vi "GUI Calibration AI.vi"(11 "error in":errorcluster) -> (15 "error out":errorcluster)   [LabVIEW 2019]
uses:
  TypeDef/CalbrationPoint.ctl
  TypeDef/GUI Setting Channel.ctl
  <vilib>/Analysis/NI_AALPro.lvlib
  <vilib>/Analysis/6fits.llb/Curve Fitting Criteria.ctl
panel:
  in  "Manual insert":bool caption="Ввод необработанного значений вручную"
  out "XY Graph - Dark":cluster{dbl[], dbl[]}[](graph) caption="Калибровачный график"
  in  "Current EU":dbl caption="Текущее значение вводится оператором"
  in  "Current RAW":dbl caption="Текущее необработанное значение"
  out "Offset":dbl caption="Смещение, EU"
  out "Коэфициент усиление":dbl caption="Коэфициент \nусиление EU/mA"
  in  "Remove Point":bool
  in  "Add Point":bool
  in  "Channels config":i32(listbox)
  in  "Channels":i32(listbox)
  # "Калибровка каналов"
  # "Параметры пересчета"
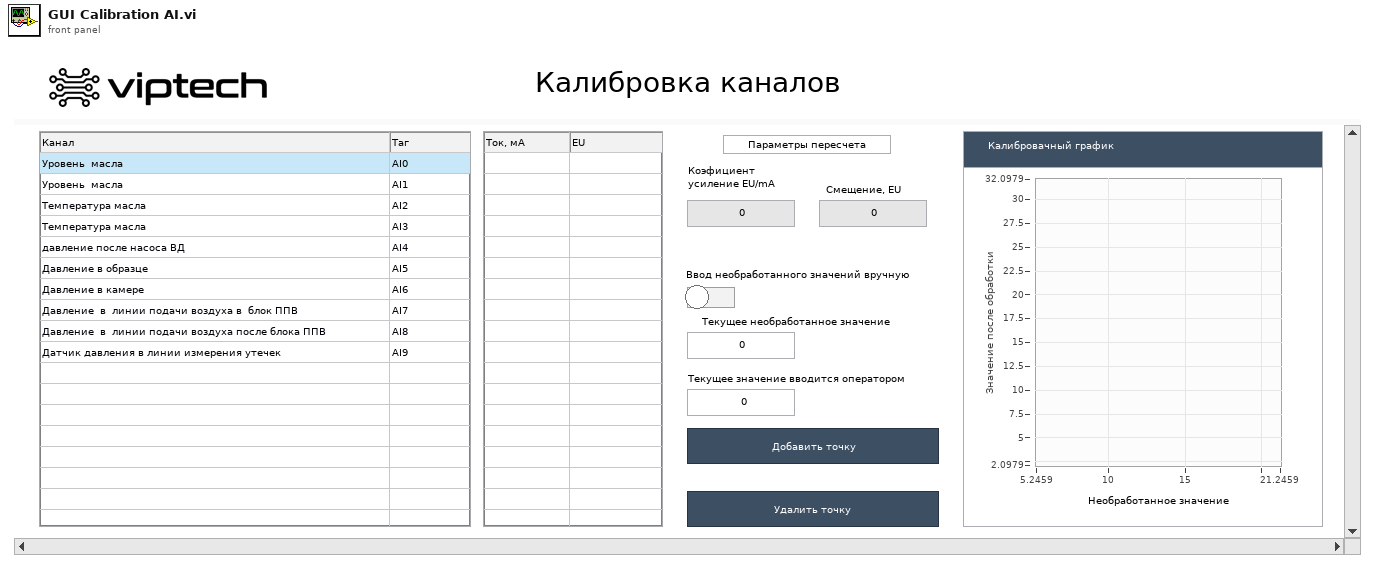
[diagram p1: front panel]
types:
  T1 = typedef "CalbrationPoint.ctl" = cluster{"RAW":dbl, "SCL":dbl}
  T2 = enum32{"Invalid", "Standard", "Closed", "Hidden", "Minimized", "Maximized"}
  T3 = enum32{"invalid app kind", "Development System", "Run Time System", "Student Edition", "Embedded LabVIEW", "Evaluation", "Custom"}
  T4 = typedef "GUI Setting Channel.ctl" = cluster{"Name":string, "SensorID":u32}
  T5 = cluster{"Core":cluster{"Current VI Reference":refnum<vi>, "Close Panel on Exit?":bool}, "Calibration Data":T4[], "Channels ref":refnum<vi>, "Channels config ref":refnum<vi>, "Channels config":i32, "Channels":i32}
  T6 = cluster{"Current VI Reference":refnum<vi>, "Close Panel on Exit?":bool}
  T7 = typedef "NI_AALPro.lvlib/Curve Fitting Criteria.ctl" = u16
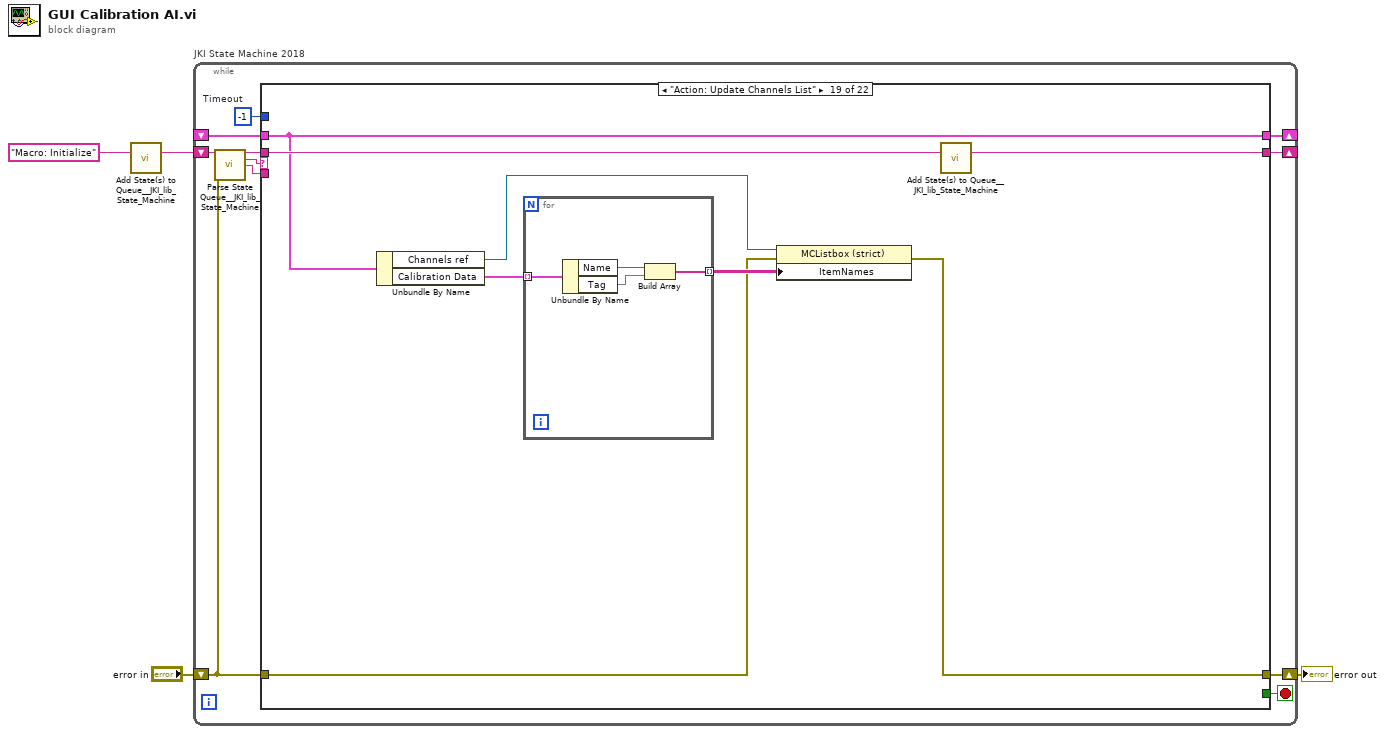
[diagram p0: block diagram]
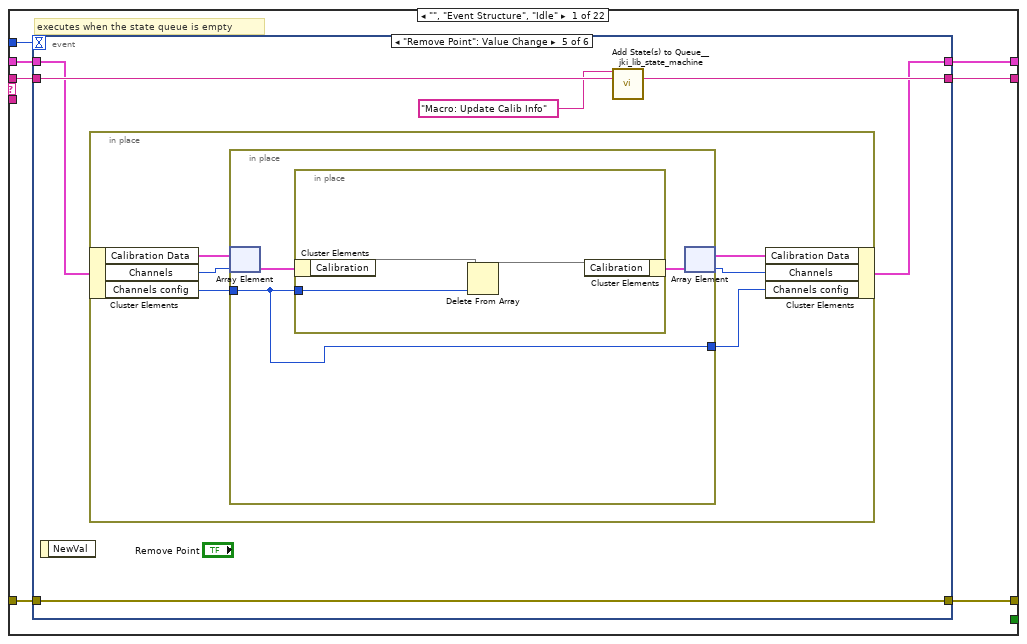
[diagram p2: hidden frame]
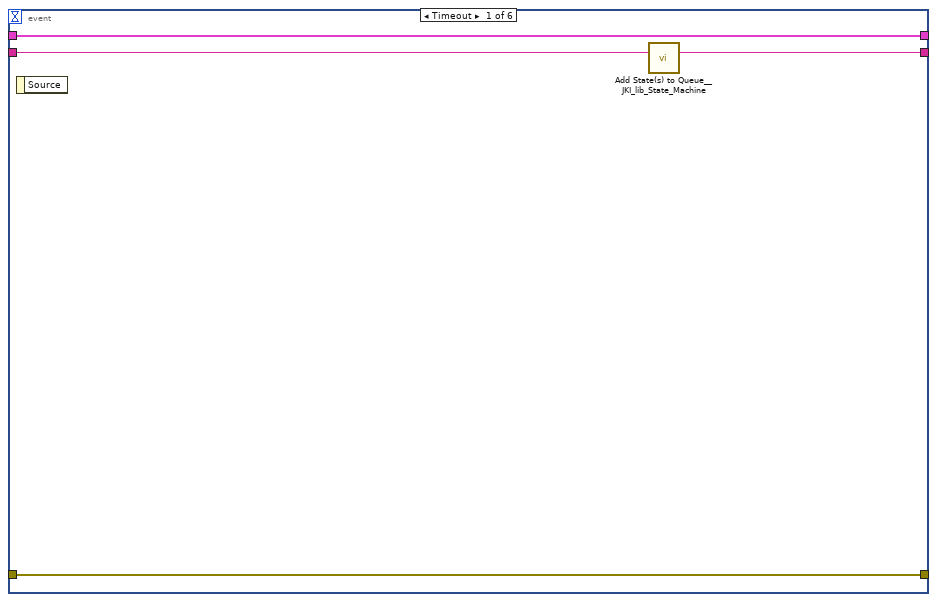
[diagram p3: hidden frame]
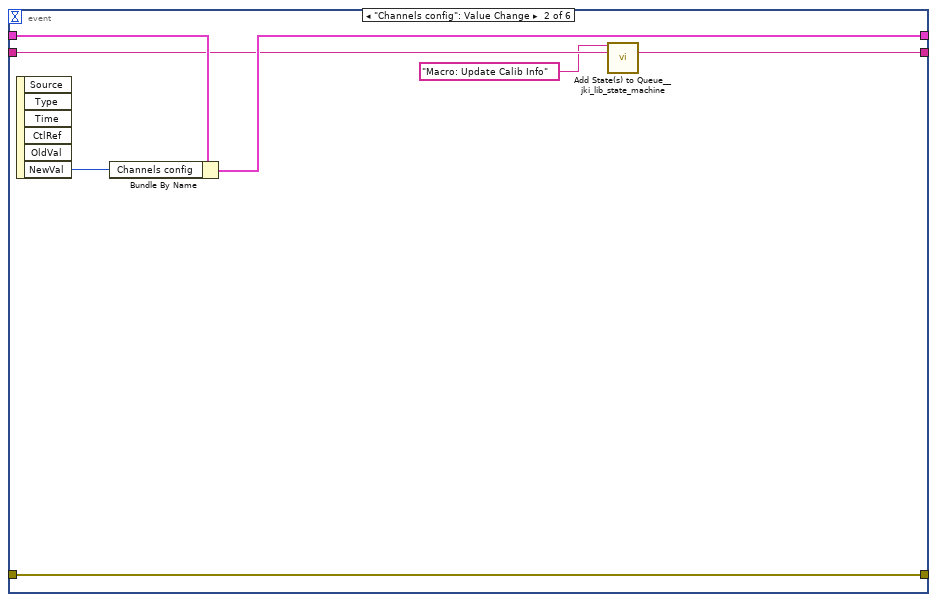
[diagram p4: hidden frame]
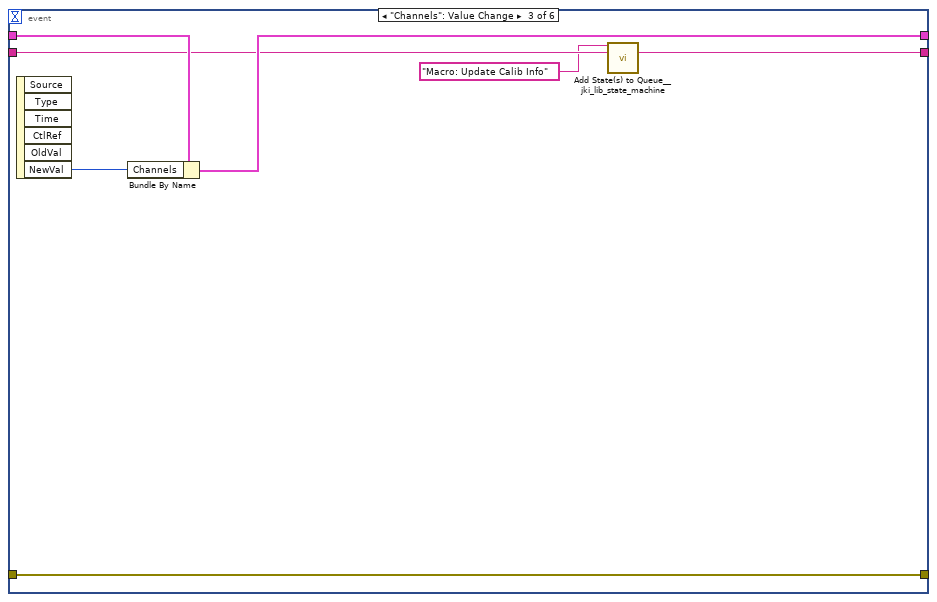
[diagram p5: hidden frame]
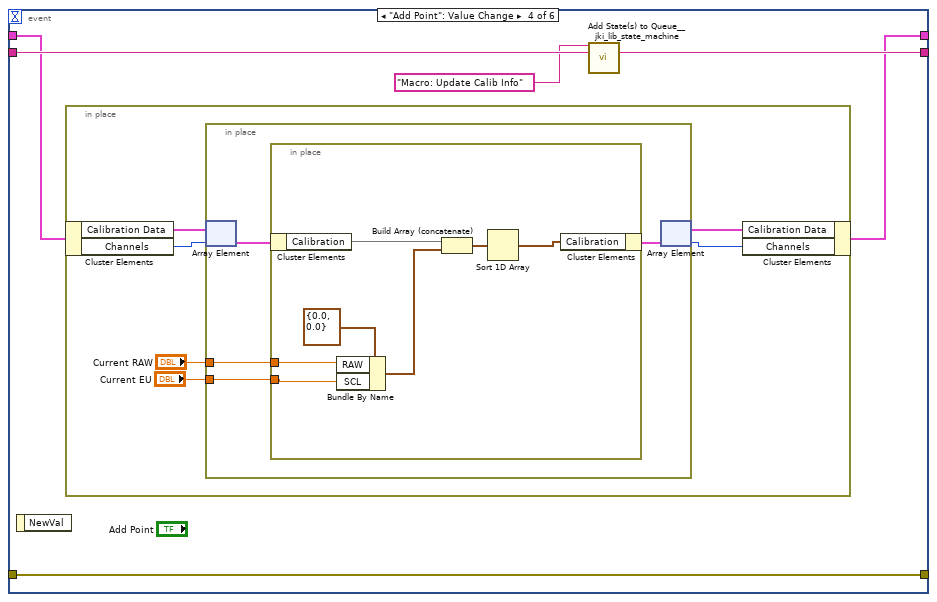
[diagram p6: hidden frame]
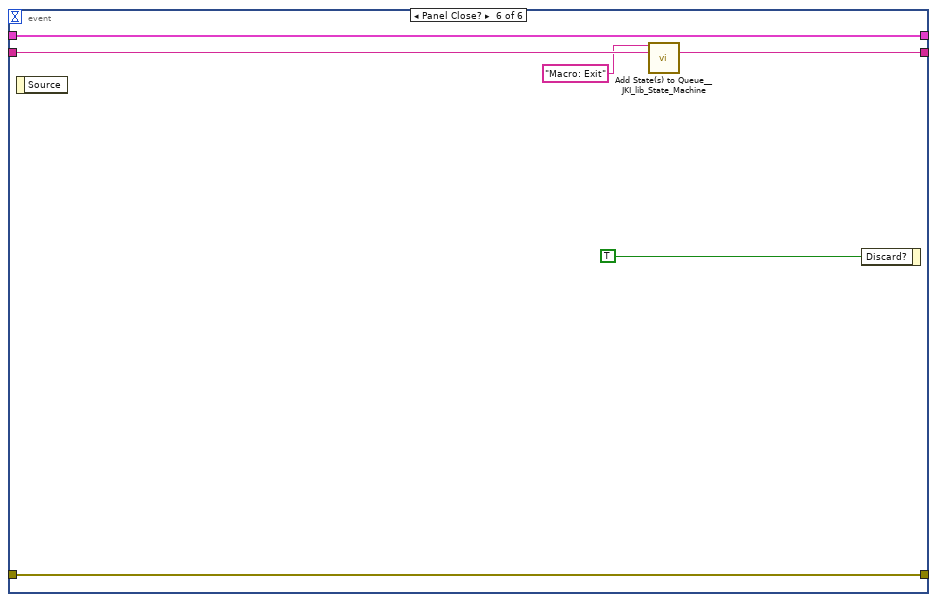
[diagram p7: hidden frame]
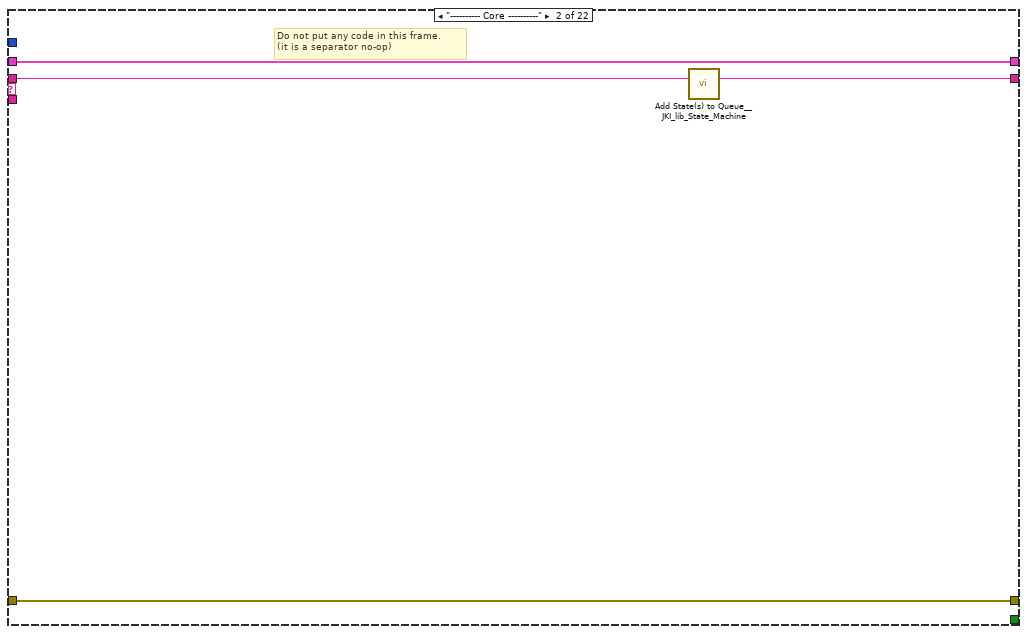
[diagram p8: hidden frame]
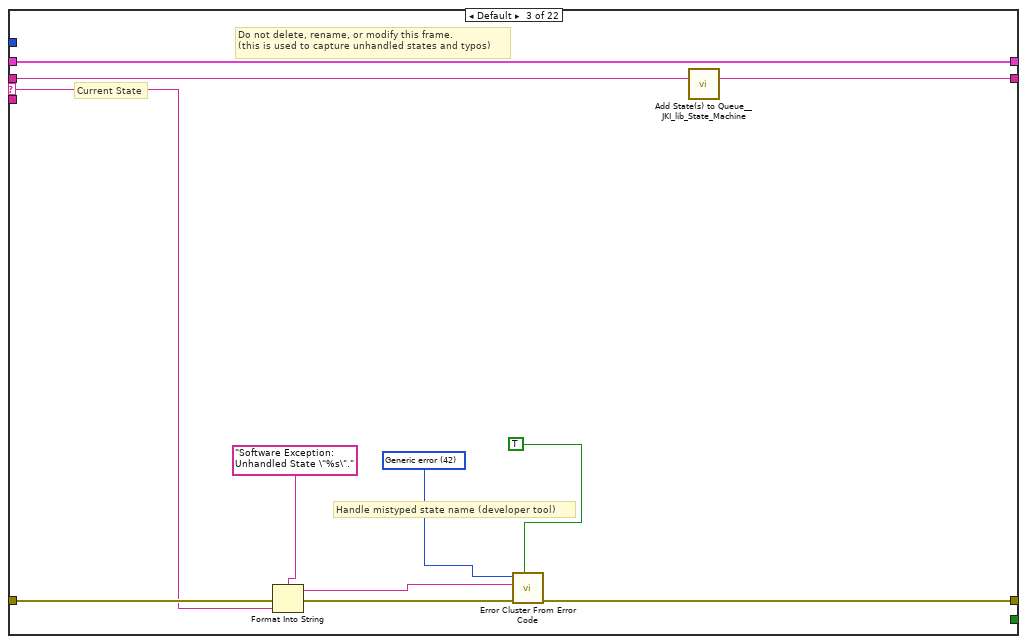
[diagram p9: hidden frame]
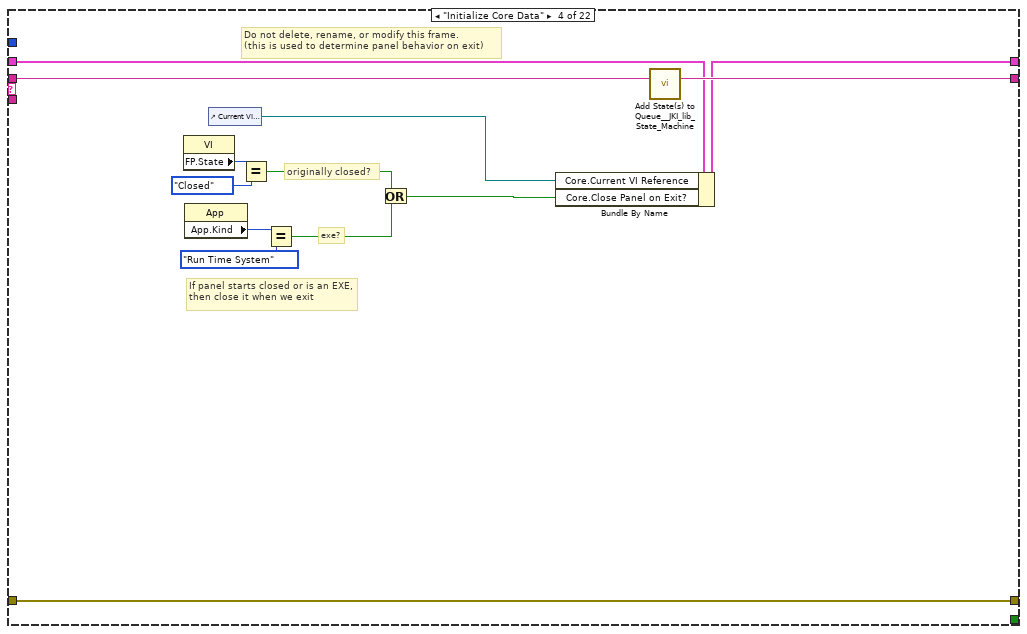
[diagram p10: hidden frame]
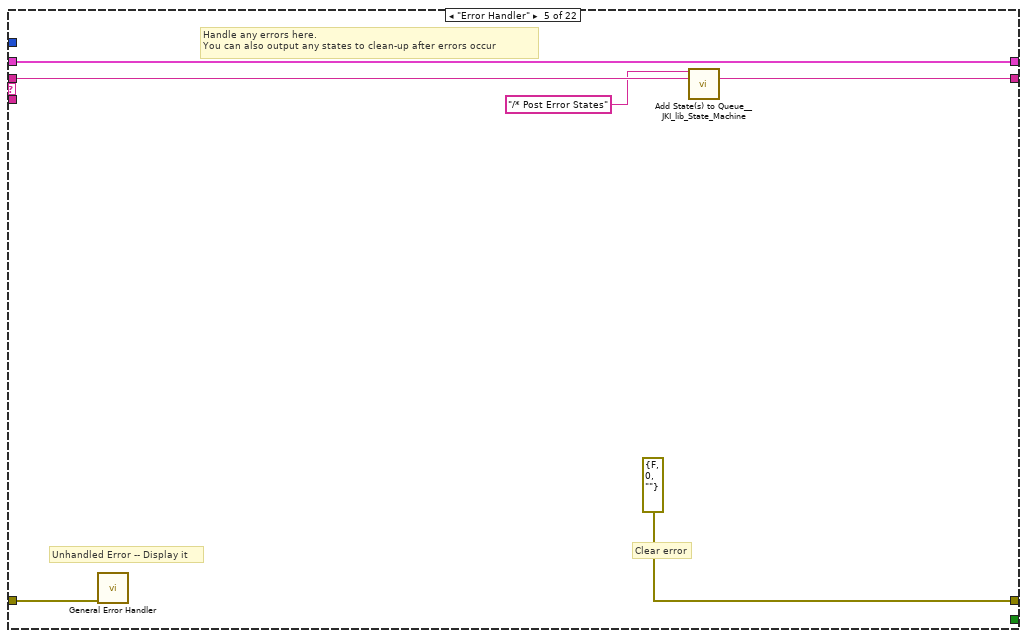
[diagram p11: hidden frame]
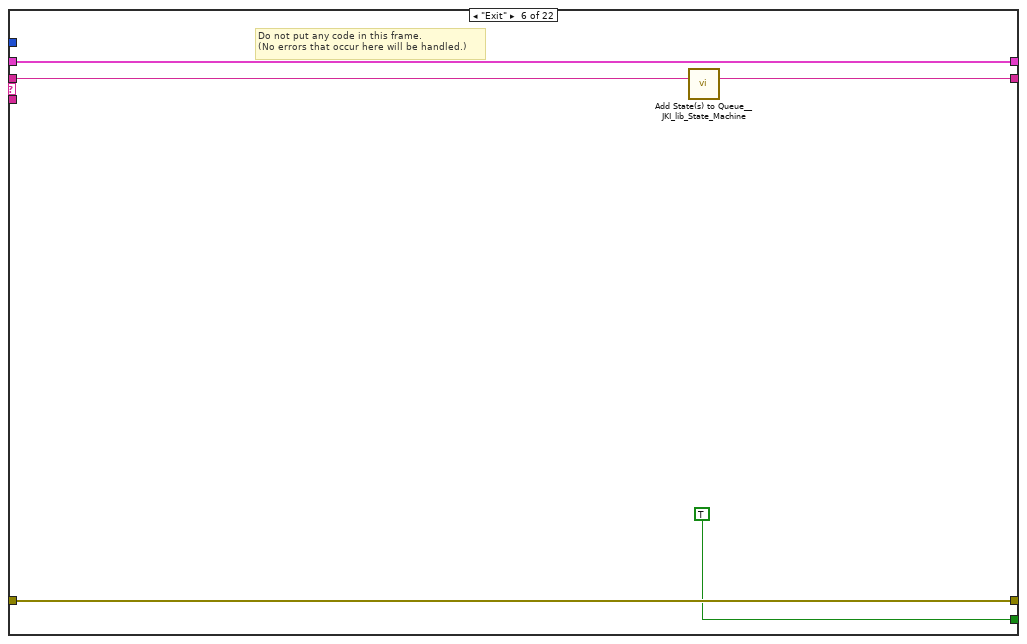
[diagram p12: hidden frame]
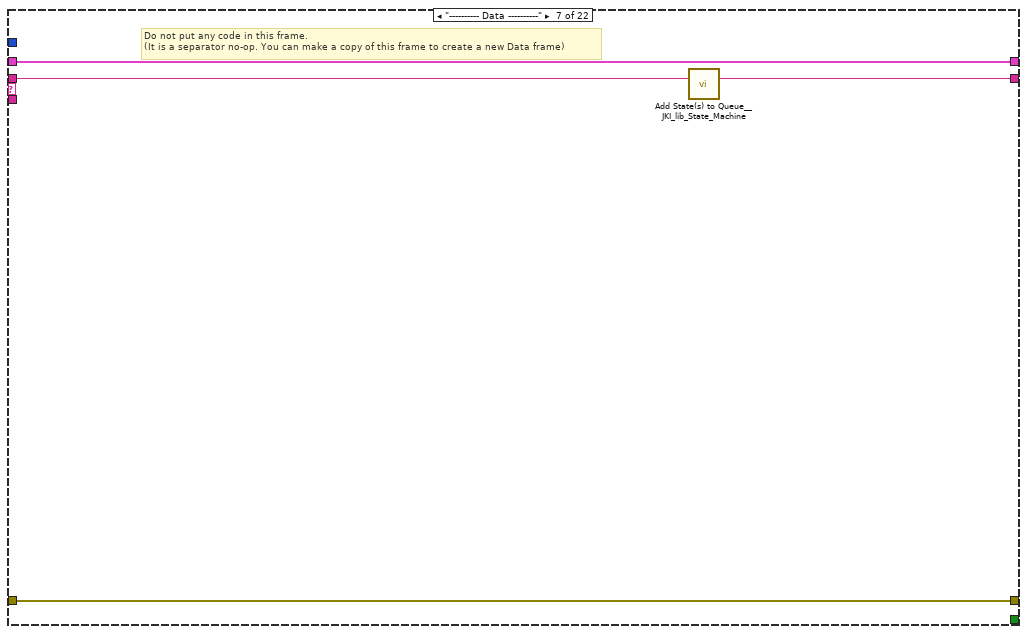
[diagram p13: hidden frame]
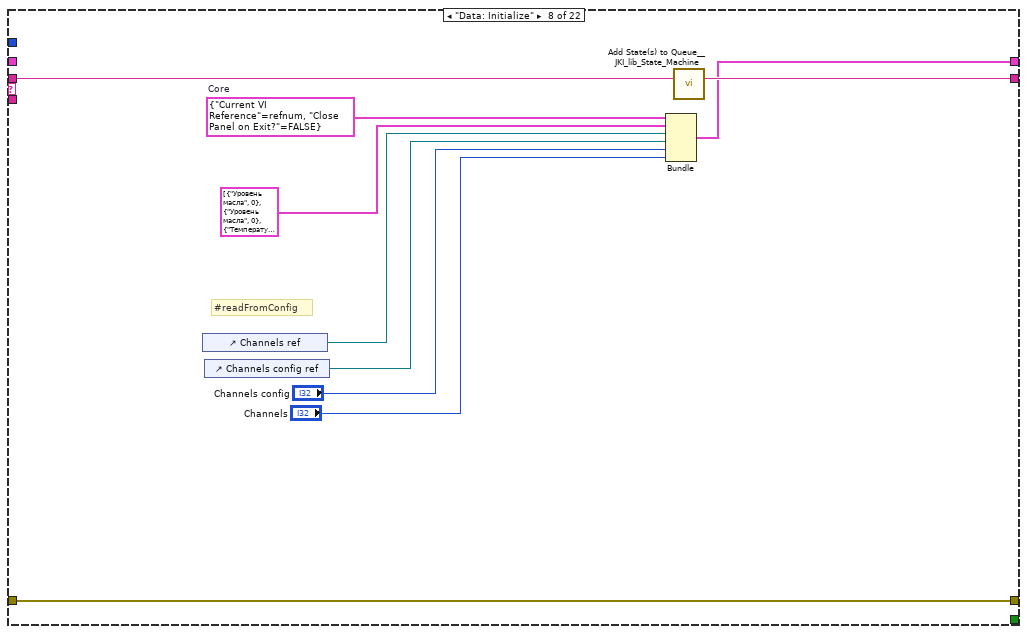
[diagram p14: hidden frame]
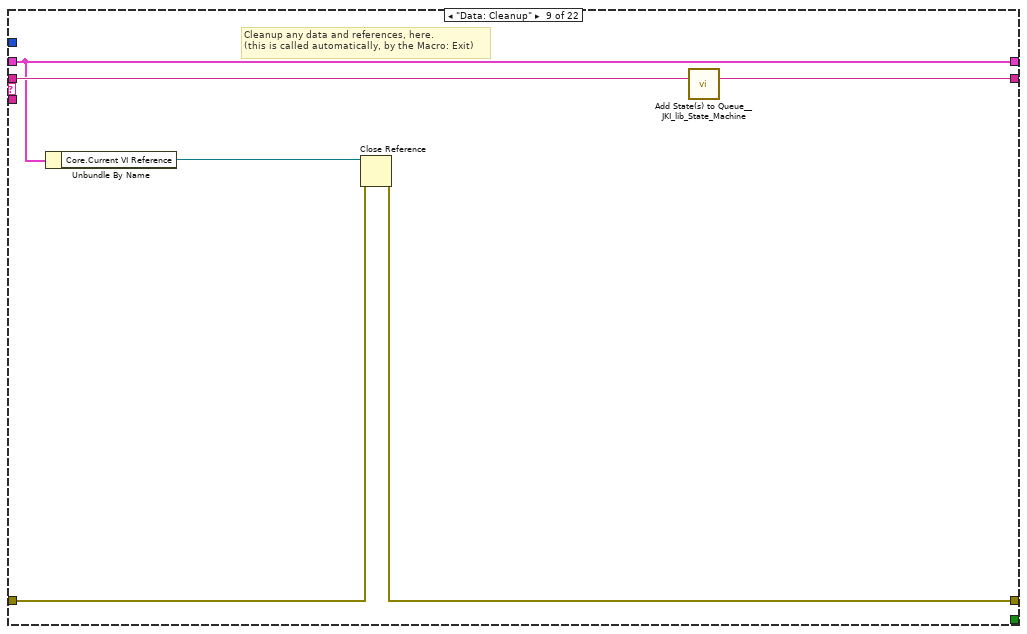
[diagram p15: hidden frame]
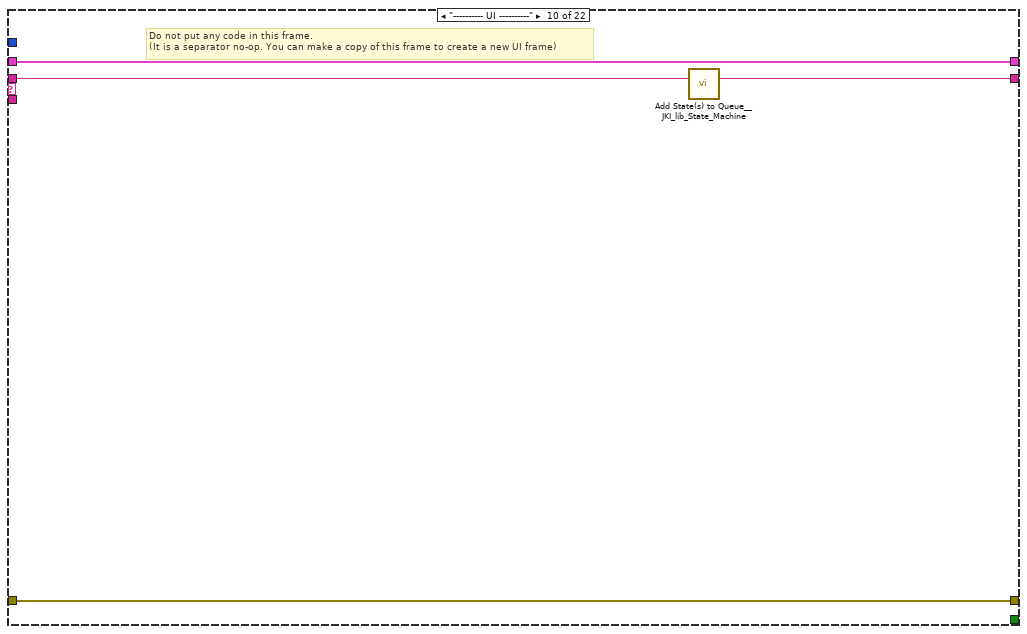
[diagram p16: hidden frame]
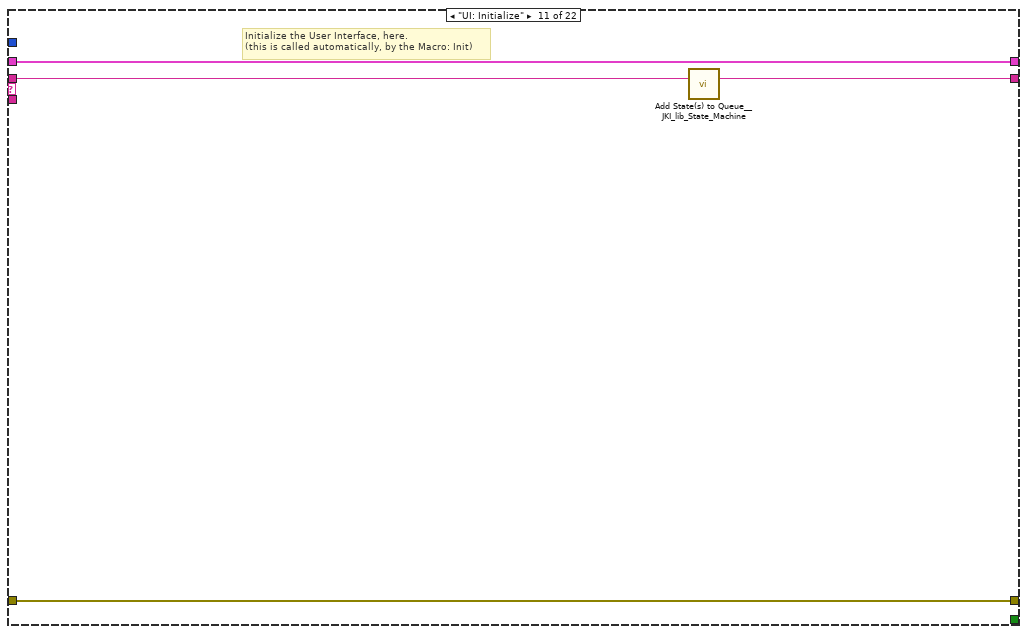
[diagram p17: hidden frame]
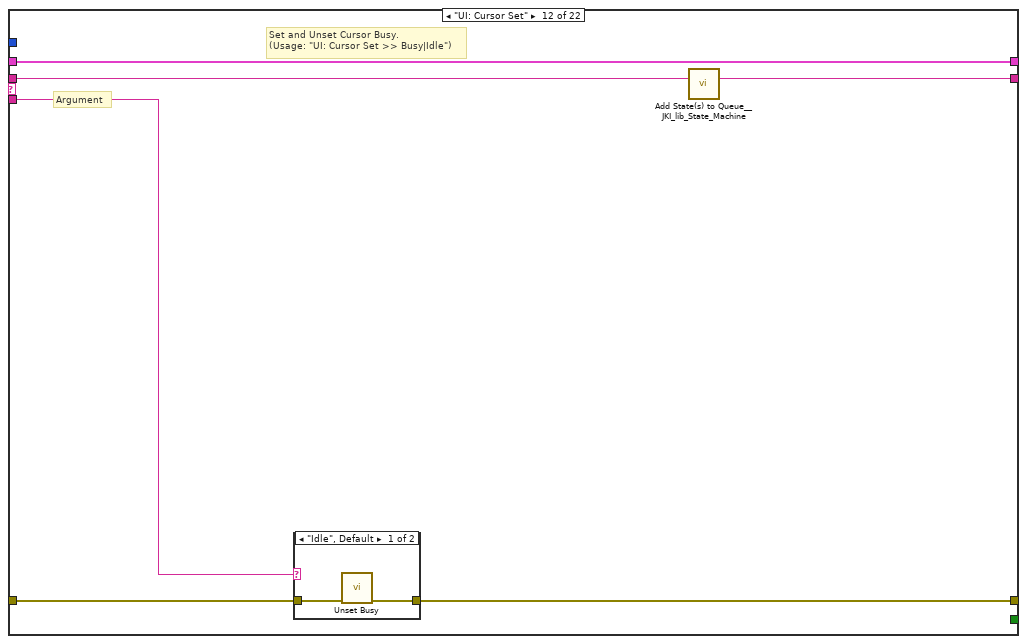
[diagram p18: hidden frame]
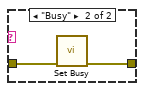
[diagram p19: hidden frame]
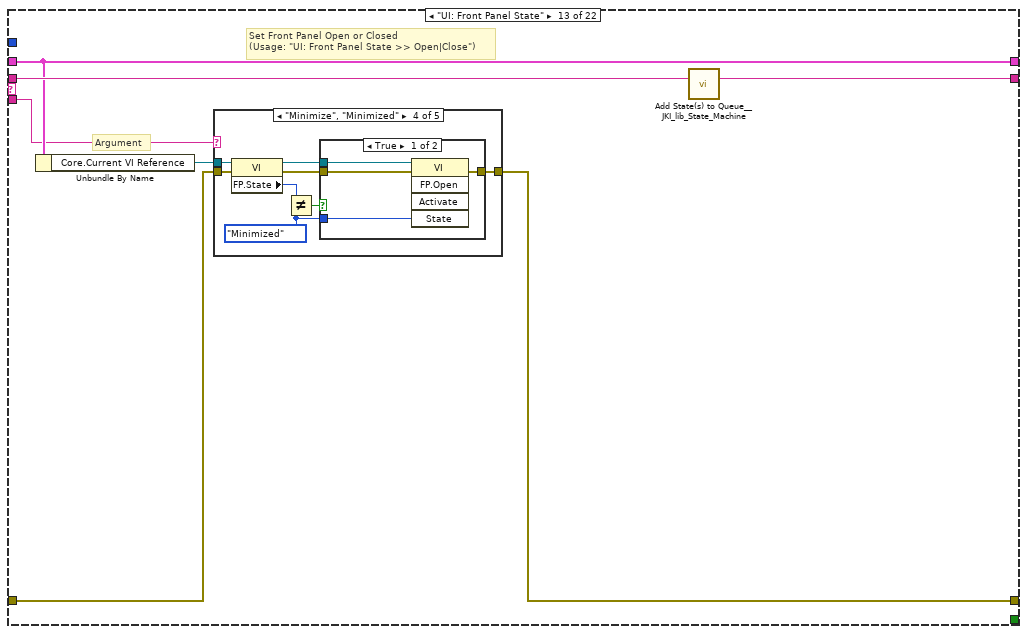
[diagram p20: hidden frame]
diagram:
  n1 = call <vilib>:"Add State(s) to Queue__JKI_lib_State_Machine.vi"("State(s) in (\"\")"="Macro: Initialize") -> ("States Out"=w4:string)  [unwired: 14 in]
  n2 = while "JKI State Machine 2018" {
    shift-right: [w8] -> _
    shift-left: _ -> [w7]
    shift-right: [w11] -> w1
    shift-left: "error in" -> [w5]
    shift-right: [w10] -> _
    shift-left: w4 -> [w12]
    stop <- w9 stop-if-true
    w6 = -1  # Timeout
    n3 = call <vilib>:"Parse State Queue__JKI_lib_State_Machine.vi"("State Queue"=w12, "Error In (no error)"=w5) -> ("Remaining States"=w14:string, "Current State"=w15:string, "Arguments"=w13:string)  [unwired: 11 in]
    n4 = case shown="\"Action: Update Channels List\"" w15 {
      selector: w15 -> [_ _ w92 _ _ _ _ _ _ _ _ _ _ _ _ _ _ _ _ _ _ _]
      tunnel: w14 -> [w22 w91 w96 w115 w121 w126 w130 w140 w146 w150 w154 w160 w171 w240 w245 w250 w260 w264 w272 w287 w300 w319]
      tunnel: w13 -> [_ _ _ _ _ _ _ _ _ _ _ w155 w165 _ _ _ _ _ _ _ _ _]
      tunnel: w7 -> [w20 w88 w94 w108 w118 w124 w127 _ w141 w147 w152 w158 w167 w237 w242 w247 w257 w261 w270 w285 w298 w316]
      tunnel: [w19 w89 w98 w112 errorcluster {"status"=FALSE, "code"=0, "source"=""} ("error out") w123 w128 w137 w142 w148 w151 w156 w168 w238 w243 w248 w258 w262 w265 w282 w299 w317] -> w11
      tunnel: w5 -> [w18 w89 w97 w112 w117 w123 w128 w137 w143 w148 w151 w157 w169 w238 w243 w248 w258 w262 w266 w283 w299 w317]
      tunnel: [w21 w90 w95 w114 w120 w125 w129 w139 w145 w149 w153 w159 w170 w239 w244 w249 w259 w263 w271 w286 w300 w318] -> w10
      tunnel: [_ _ _ _ _ TRUE _ _ _ _ _ _ _ _ _ _ _ _ _ _ _ _] -> w9
      tunnel: [w17 w88 w94 w113 w118 w124 w127 w138 w141 w147 w152 w158 w167 w237 w242 w247 w257 w261 w270 w285 w295 w316] -> w8
      tunnel: w6 -> [w16 _ _ _ _ _ _ _ _ _ _ _ _ _ _ _ _ _ _ _ _ _]
      frame "", "Event Structure", "Idle" {
        # "executes when the state queue is empty"
        n5 = event shown="[4] \"Remove Point\": Value Change" {
          selector: _ -> [_ _ _ _ _ _]
          dyn-events: _ -> [_ _ _ _ _ _]
          timeout: w16 -> [_ _ _ _ _ _]
          tunnel: w22 -> [w26 w28 w35 w44 w67 w87]
          tunnel: [w25 w29 w36 w45 w68 w86] -> w21
          tunnel: w20 -> [w23 w33 w40 w42 w65 w84]
          tunnel: [w24 w32 w39 w46 w69 w85] -> w19
          tunnel: w18 -> [w24 w32 w39 w46 w69 w85]
          tunnel: [w23 w31 w38 w41 w64 w84] -> w17
          event Timeout {
            n6 = event-data() -> ()  [unwired: 1 in, 1 out]
            n7 = call <vilib>:"Add State(s) to Queue__JKI_lib_State_Machine.vi"("State(s) in (\"\")"=w26) -> ("States Out"=w25:string)  [unwired: 14 in]
          }
          event "Channels config": Value Change {
            n8 = event-data() -> ("NewVal"=w30:i32)  [unwired: 1 in, 5 out]
            n9 = Bundle By Name(cluster=w33, "Channels config"=w30) -> (w31:T5)
            n10 = call <vilib>:"Add State(s) to Queue__jki_lib_state_machine.vi"("State(s) in Front (\"\")"="Macro: Update Calib Info" ("State(s) in Front (\"\")"), "State(s) in (\"\")"=w28) -> ("States Out"=w29:string)  [unwired: 13 in]
          }
          event "Channels": Value Change {
            n11 = event-data() -> ("NewVal"=w37:i32)  [unwired: 1 in, 5 out]
            n12 = Bundle By Name(cluster=w40, "Channels"=w37) -> (w38:T5)
            n13 = call <vilib>:"Add State(s) to Queue__jki_lib_state_machine.vi"("State(s) in Front (\"\")"="Macro: Update Calib Info" ("State(s) in Front (\"\")"), "State(s) in (\"\")"=w35) -> ("States Out"=w36:string)  [unwired: 13 in]
          }
          event "Add Point": Value Change {
            n14 = event-data() -> ()  [unwired: 1 in, 1 out]
            n15 = in-place {
              n16 = in-place-cluster #1(w42) -> ("Calibration Data"=w52:T4[], "Channels"=w51:i32)
              n17 = in-place {
                in-place-border: "Current EU" -> [w55]
                in-place-border: "Current RAW" -> [w54]
                n18 = in-place-array #2(w52, w51) -> (w56:T4)
                n19 = in-place {
                  in-place-border: w55 -> [w59]
                  in-place-border: w54 -> [w60]
                  n20 = in-place-cluster #3(w56) -> ("Calibration"=w63)
                  n21 = Bundle By Name(cluster=T1 {"RAW"=0.0, "SCL"=0.0} ("Point"), "RAW"=w60, "SCL"=w59) -> (w61:T1)
                  n22 = Build Array (concatenate)(w63, w61) -> (w58:T1[])
                  n23 = Sort 1D Array(array=w58) -> (sorted array=w57:T1[])
                  n24 = in-place-cluster #3("Calibration"=w57) -> (w53:T4)
                }
                n25 = in-place-array #2(w53) -> (w50:T4[], w49:i32)
              }
              n26 = in-place-cluster #1("Calibration Data"=w50, "Channels"=w49) -> (w41:T5)
            }
            n27 = call <vilib>:"Add State(s) to Queue__jki_lib_state_machine.vi"("State(s) in Front (\"\")"="Macro: Update Calib Info" ("State(s) in Front (\"\")"), "State(s) in (\"\")"=w44) -> ("States Out"=w45:string)  [unwired: 13 in]
          }
          event "Remove Point": Value Change {
            n28 = event-data() -> ()  [unwired: 1 in, 1 out]
            n29 = in-place {
              n30 = in-place-cluster #4(w65) -> ("Calibration Data"=w75:T4[], "Channels"=w74:i32, "Channels config"=w71:i32)
              n31 = in-place {
                in-place-border: w71 -> [w76]
                in-place-border: [w76] -> w70
                n32 = in-place-array #5(w75, w74) -> (w78:T4)
                n33 = in-place {
                  in-place-border: w76 -> [w79]
                  n34 = in-place-cluster #6(w78) -> ("Calibration"=w81)
                  n35 = Delete From Array(array=w81, index=w79) -> (array with subset deleted=w80)  [unwired: 1 in, 1 out]
                  n36 = in-place-cluster #6("Calibration"=w80) -> (w77:T4)
                }
                n37 = in-place-array #5(w77) -> (w73:T4[], w72:i32)
              }
              n38 = in-place-cluster #4("Calibration Data"=w73, "Channels"=w72, "Channels config"=w70) -> (w64:T5)
            }
            n39 = call <vilib>:"Add State(s) to Queue__jki_lib_state_machine.vi"("State(s) in Front (\"\")"="Macro: Update Calib Info" ("State(s) in Front (\"\")"), "State(s) in (\"\")"=w67) -> ("States Out"=w68:string)  [unwired: 13 in]
          }
          event Panel Close? {
            n40 = event-data() -> ()  [unwired: 1 in, 1 out]
            n41 = call <vilib>:"Add State(s) to Queue__JKI_lib_State_Machine.vi"("State(s) in Front (\"\")"="Macro: Exit", "State(s) in (\"\")"=w87) -> ("States Out"=w86:string)  [unwired: 13 in]
            n42 = event-data("Discard?"=TRUE) -> ()  [unwired: 1 in, 1 out]
          }
        }
      }
      frame "---------- Core ----------" {
        # "Do not put any code in this frame.\n(it is a separator no-op)"
        n43 = call <vilib>:"Add State(s) to Queue__JKI_lib_State_Machine.vi"("State(s) in (\"\")"=w91) -> ("States Out"=w90:string)  [unwired: 14 in]
      }
      frame Default {
        w101 = 42 items=["No error", "Argument error", "Memory is full", "Out of zone", "End of file", "File already open", "Generic file I/O error", "File not found", "File permission error", "Disk is full", "Duplicate path", "Too many files open", "System feature not enabled", "Resource file not found", "Cannot add resource", "Resource not found", "Image not found", "Image memory error", "Pen does not exist", "Config type invalid", "Config token not found", "Config parse error", "Config memory error", "Bad external code format", "Bad external code offset", "External code not present", "Null window", "Destroy window error", "Null menu", "Print aborted", "Bad print record", "Print driver error", "Windows error during printing", "Memory error during printing", "Print dialog error", "Generic print error", "Invalid device refnum", "Device not found", "Device parameter error", "Device unit error", "Cannot open device", "Device call aborted", "Generic error", "Cancelled by user", "Object ID too low", "Object ID too high", "Object not in heap", "Unknown heap", "Unknown object (invalid DefProc)", "Unknown object (DefProc not in table)", "Message out of range", "Invalid (null) method", "Unknown message", "Manager call not supported", "Bad address", "Network operation in progress", "Network operation timed out", "Connection is busy", "Network attribute not supported", "Network error", "Address in use", "System out of memory", "Connection aborted", "Connection refused", "Not connected", "Already connected", "Connection closed", "Initialization error (interapplication manager)", "Bad occurrence", "Wait on unbound occurrence handler", "Occurrence queue overflow", "Datalog type conflict", "Unused", "Unrecognized type (interapplication manager)", "Memory corrupt", "Failed to make temporary DLL", "Old CIN version", "Drag socket not found", "Failed to load drop-object", "Failed to register OLE object", "Failed to release OLE object", "Format specifier type mismatch", "Unknown format specifier", "Too few format specifiers", "Too many format specifiers", "Scan failed", "Newer CIN version", "Error converting to variant", "Runtime menu error", "Password tampered", "Variant attribute not found", "Incompatible variant data type", "Event data is not available", "Event Store is not present", "Occurrence is not found", "Event Queue is not created", "Event info is not available", "Refnum passed is NULL", "Error retrieving Class GUID", "Error retrieving CoClass GUID", "Error retrieving TypeLib GUID.", "Bad built application magic bytes.", "Specific driver is different from the specific driver associated with the Logical Name.", "There is no session opened to the class driver.", "Max Error", "MAX - Error with config objects", "MAX - Error loading configuration", "MAX - Group not supported"]
        # "Current State"
        # "Do not delete, rename, or modify this frame.\n(this is used to capture unhandled states and typos)"
        # "Handle mistyped state name (developer tool)"
        n44 = Format Into String(format string="Software Exception: Unhandled State \"%s\"." ("message"), error in=w97, w92) -> (resulting string=w100:string, error out=w99:errorcluster)  [unwired: 1 in]
        n45 = call <vilib>:"Error Cluster From Error Code.vi"("show call chain? (False)"=TRUE, "error in (no error)"=w99, "error message (\"\")"=w100, "error code (0)"=w101) -> ("error out"=w98:errorcluster)  [unwired: 5 in]
        n46 = call <vilib>:"Add State(s) to Queue__JKI_lib_State_Machine.vi"("State(s) in (\"\")"=w96) -> ("States Out"=w95:string)  [unwired: 14 in]
      }
      frame "Initialize Core Data" {
        # "Do not delete, rename, or modify this frame.\n(this is used to determine panel behavior on exit)"
        # "originally closed?"
        # "exe?"
        # "If panel starts closed or is an EXE, then close it when we exit"
        n47 = property class="VI"() -> ("FP.State"=w105:T2)  [unwired: 2 in, 2 out]
        n48 = property class="App"() -> ("App.Kind"=w111:T3)  [unwired: 2 in, 2 out]
        n49 = control-ref of="Current VI Reference"() -> (w106:refnum<vi>)
        n50 = Equal?(x=w105, y=T2."Closed" ("Front Panel Window:State")) -> (x = y?=w103:bool)
        n51 = Equal?(x=w111, y=T3."Run Time System" ("Application:Kind")) -> (x = y?=w109:bool)
        n52 = Or(x=w103, y=w109) -> (x .or. y?=w107:bool)
        n53 = Bundle By Name(cluster=w108, "Core.Current VI Reference"=w106, "Core.Close Panel on Exit?"=w107) -> (w113:T5)
        n54 = call <vilib>:"Add State(s) to Queue__JKI_lib_State_Machine.vi"("State(s) in (\"\")"=w115) -> ("States Out"=w114:string)  [unwired: 14 in]
      }
      frame "Error Handler" {
        # "Unhandled Error -- Display it"
        # "Handle any errors here.\nYou can also output any states to clean-up after errors occur"
        # "Clear error"
        n55 = call <vilib>:"General Error Handler.vi"("error in (no error)"=w117) -> ()  [unwired: 10 in, 5 out]
        n56 = call <vilib>:"Add State(s) to Queue__JKI_lib_State_Machine.vi"("State(s) in Front (\"\")"="/* Post Error States", "State(s) in (\"\")"=w121) -> ("States Out"=w120:string)  [unwired: 13 in]
      }
      frame "Exit" {
        # "Do not put any code in this frame.\n(No errors that occur here will be handled.)"
        n57 = call <vilib>:"Add State(s) to Queue__JKI_lib_State_Machine.vi"("State(s) in (\"\")"=w126) -> ("States Out"=w125:string)  [unwired: 14 in]
      }
      frame "---------- Data ----------" {
        # "Do not put any code in this frame.\n(It is a separator no-op. You can make a copy of this frame to create a new Data frame)"
        n58 = call <vilib>:"Add State(s) to Queue__JKI_lib_State_Machine.vi"("State(s) in (\"\")"=w130) -> ("States Out"=w129:string)  [unwired: 14 in]
      }
      frame "Data: Initialize" {
        w136 = T6 {"Current VI Reference"=refnum, "Close Panel on Exit?"=FALSE}  # Core
        # "#readFromConfig"
        n59 = control-ref of="Channels ref"() -> (w134:refnum<vi>)
        n60 = control-ref of="Channels config ref"() -> (w133:refnum<vi>)
        n61 = Bundle("Core"=w136, "Calibration Data"=T4[] [{"Name"="Уровень  масла", "SensorID"=0}, {"Name"="Уровень  масла", "SensorID"=0}, {"Name"="Температура масла", "SensorID"=0}, {"Name"="Температура масла", "SensorID"=0}, {"Name"="давление после насоса ВД", "SensorID"=0}, {"Name"="Давление в образце", "SensorID"=0}, {"Name"="Давление в камере", "SensorID"=0}, {"Name"="Давление  в  линии подачи воздуха в  блок ППВ", "SensorID"=0}, {"Name"="Давление  в  линии подачи воздуха после блока ППВ", "SensorID"=0}, {"Name"="Датчик давления в линии измерения утечек", "SensorID"=0}], "Channels ref"=w134, "Channels config ref"=w133, "Channels config"="Channels config", "Channels"="Channels") -> (w138:T5)  [unwired: 1 in]
        n62 = call <vilib>:"Add State(s) to Queue__JKI_lib_State_Machine.vi"("State(s) in (\"\")"=w140) -> ("States Out"=w139:string)  [unwired: 14 in]
      }
      frame "Data: Cleanup" {
        # "Cleanup any data and references, here.\n(this is called automatically, by the Macro: Exit)"
        n63 = Unbundle By Name(w141) -> ("Core.Current VI Reference"=w144:refnum<vi>)
        n64 = Close Reference(reference=w144, error in (no error)=w143) -> (error out=w142:errorcluster)
        n65 = call <vilib>:"Add State(s) to Queue__JKI_lib_State_Machine.vi"("State(s) in (\"\")"=w146) -> ("States Out"=w145:string)  [unwired: 14 in]
      }
      frame "---------- UI ----------" {
        # "Do not put any code in this frame.\n(It is a separator no-op. You can make a copy of this frame to create a new UI frame)"
        n66 = call <vilib>:"Add State(s) to Queue__JKI_lib_State_Machine.vi"("State(s) in (\"\")"=w150) -> ("States Out"=w149:string)  [unwired: 14 in]
      }
      frame "UI: Initialize" {
        # "Initialize the User Interface, here.\n(this is called automatically, by the Macro: Init)"
        n67 = call <vilib>:"Add State(s) to Queue__JKI_lib_State_Machine.vi"("State(s) in (\"\")"=w154) -> ("States Out"=w153:string)  [unwired: 14 in]
      }
      frame "UI: Cursor Set" {
        # "Argument"
        # "Set and Unset Cursor Busy.\n(Usage: \"UI: Cursor Set >> Busy|Idle\")"
        n68 = case shown="\"Idle\", Default" w155 {
          tunnel: w157 -> [w162 w164]
          tunnel: [w161 w163] -> w156
          frame "Idle", Default {
            n69 = call <vilib>:"Unset Busy.vi"("error in (no error)"=w162) -> ("error out"=w161:errorcluster)  [unwired: 10 in]
          }
          frame "Busy" {
            n70 = call <vilib>:"Set Busy.vi"("error in (no error)"=w164) -> ("error out"=w163:errorcluster)  [unwired: 9 in, 1 out]
          }
        }
        n71 = call <vilib>:"Add State(s) to Queue__JKI_lib_State_Machine.vi"("State(s) in (\"\")"=w160) -> ("States Out"=w159:string)  [unwired: 14 in]
      }
      frame "UI: Front Panel State" {
        # "Argument"
        # "Set Front Panel Open or Closed\n(Usage: \"UI: Front Panel State >> Open|Close\")"
        n72 = Unbundle By Name(w167) -> ("Core.Current VI Reference"=w166:refnum<vi>)
        n73 = case shown="\"Minimize\", \"Minimized\"" w165 {
          tunnel: w169 -> [w177 w192 w203 w216 w229]
          tunnel: [w179 w193 w205 w218 w231] -> w168
          tunnel: w166 -> [w178 w190 w204 w217 w230]
          frame "Open", "Standard", Default {
            w172 = T2."Standard" ("State")
            n74 = property class="VI"(reference=w178, error in=w177) -> (reference out=w175:refnum<vi>, error out=w176:errorcluster, "FP.State"=w174:T2)
            n75 = Not Equal?(x=w174, y=w172) -> (x != y?=w173:bool)
            n76 = case shown="True" w173 {
              tunnel: [w183 w185] -> w179
              tunnel: w176 -> [w182 w185]
              tunnel: w175 -> [w181 _]
              tunnel: w172 -> [w180 _]
              frame True {
                n77 = invoke class="VI" method="FP.Open"(reference=w181, error in=w182, "Activate"=TRUE, "State"=w180) -> (error out=w183:errorcluster)  [unwired: 1 in, 4 out]
              }
              frame False {
              }
            }
          }
          frame "Close", "Closed" {
            n78 = property class="VI"(reference=w190, error in=w192) -> (reference out=w189:refnum<vi>, error out=w191:errorcluster, "FP.State"=w187:T2)
            n79 = Not Equal?(x=w187, y=T2."Closed" ("Front Panel Window:State")) -> (x != y?=w186:bool)
            n80 = case shown="True" w186 {
              tunnel: [w194 w197] -> w193
              tunnel: w191 -> [w194 w196]
              tunnel: w189 -> [_ w195]
              frame False {
              }
              frame True {
                n81 = invoke class="VI" method="FP.Close"(reference=w195, error in=w196) -> (error out=w197:errorcluster)  [unwired: 1 in, 2 out]
              }
            }
          }
          frame "Hidden", "Hide" {
            w198 = T2."Hidden" ("State")
            n82 = property class="VI"(reference=w204, error in=w203) -> (reference out=w201:refnum<vi>, error out=w202:errorcluster, "FP.State"=w200:T2)
            n83 = Not Equal?(x=w200, y=w198) -> (x != y?=w199:bool)
            n84 = case shown="True" w199 {
              tunnel: [w209 w210] -> w205
              tunnel: w202 -> [w208 w210]
              tunnel: w201 -> [w207 _]
              tunnel: w198 -> [w206 _]
              frame True {
                n85 = invoke class="VI" method="FP.Open"(reference=w207, error in=w208, "State"=w206) -> (error out=w209:errorcluster)  [unwired: 2 in, 4 out]
              }
              frame False {
              }
            }
          }
          frame "Minimize", "Minimized" {
            w211 = T2."Minimized" ("State")
            n86 = property class="VI"(reference=w217, error in=w216) -> (reference out=w214:refnum<vi>, error out=w215:errorcluster, "FP.State"=w213:T2)
            n87 = Not Equal?(x=w213, y=w211) -> (x != y?=w212:bool)
            n88 = case shown="True" w212 {
              tunnel: [w222 w223] -> w218
              tunnel: w215 -> [w221 w223]
              tunnel: w214 -> [w220 _]
              tunnel: w211 -> [w219 _]
              frame True {
                n89 = invoke class="VI" method="FP.Open"(reference=w220, error in=w221, "State"=w219) -> (error out=w222:errorcluster)  [unwired: 2 in, 4 out]
              }
              frame False {
              }
            }
          }
          frame "Maximize", "Maximized" {
            w224 = T2."Maximized" ("State")
            n90 = property class="VI"(reference=w230, error in=w229) -> (reference out=w227:refnum<vi>, error out=w228:errorcluster, "FP.State"=w226:T2)
            n91 = Not Equal?(x=w226, y=w224) -> (x != y?=w225:bool)
            n92 = case shown="True" w225 {
              tunnel: [w235 w236] -> w231
              tunnel: w228 -> [w234 w236]
              tunnel: w227 -> [w233 _]
              tunnel: w224 -> [w232 _]
              frame True {
                n93 = invoke class="VI" method="FP.Open"(reference=w233, error in=w234, "State"=w232) -> (error out=w235:errorcluster)  [unwired: 2 in, 4 out]
              }
              frame False {
              }
            }
          }
        }
        n94 = call <vilib>:"Add State(s) to Queue__JKI_lib_State_Machine.vi"("State(s) in (\"\")"=w171) -> ("States Out"=w170:string)  [unwired: 14 in]
      }
      frame "---------- Macro ----------" {
        # "Do not put any code in this frame.\n(It is a separator no-op. You can make a copy of this frame to create a new Macro frame)"
        n95 = call <vilib>:"Add State(s) to Queue__JKI_lib_State_Machine.vi"("State(s) in (\"\")"=w240) -> ("States Out"=w239:string)  [unwired: 14 in]
      }
      frame "Macro: Update Calib Info" {
        # "Do not put any code in this frame.\n(It is a separator no-op. You can make a copy of this frame to create a new Macro frame)"
        n96 = call <vilib>:"Add State(s) to Queue__JKI_lib_State_Machine.vi"("State(s) in Front (\"\")"="Action: Update Calibration Tbl\nAction: Update Calib Graph", "State(s) in (\"\")"=w245) -> ("States Out"=w244:string)  [unwired: 13 in]
      }
      frame "Macro: Initialize" {
        w246 = "Data: Initialize\nInitialize Core Data\nUI: Initialize\nUI: Front Panel State >> Open\n\n\n\nAction: Update Channels List\nMacro: Update Calib Info"  # Data: Initialize Initialize Core Data UI: Initialize UI: Front Panel State >> Open    Action: Update Channels List Macro: Update Calib Info
        n97 = call <vilib>:"Add State(s) to Queue__JKI_lib_State_Machine.vi"("State(s) in Front (\"\")"=w246, "State(s) in (\"\")"=w250) -> ("States Out"=w249:string)  [unwired: 13 in]
      }
      frame "Macro: Exit" {
        # "Exit Macro\n(This is called once, when the VI exits)"
        n98 = Unbundle By Name(w257) -> ("Core.Close Panel on Exit?"=w256:bool)
        n99 = Select(t="UI: Front Panel State >> Close", s=w256, f="") -> (s? t:f=w253:string)
        n100 = call <vilib>:"Add State(s) to Queue__JKI_lib_State_Machine.vi"("State(s) in (\"\")"=w253, "State(s) at Back (\"\")"="Data: Cleanup\nExit") -> ("States Out"=w251:string)  [unwired: 13 in]
        n101 = call <vilib>:"Add State(s) to Queue__JKI_lib_State_Machine.vi"("State(s) in Front (\"\")"=w251, "State(s) in (\"\")"=w260) -> ("States Out"=w259:string)  [unwired: 13 in]
      }
      frame "---------- Action ----------" {
        # "Template Separator\n(You can make a copy of, or modify, this frame)"
        n102 = call <vilib>:"Add State(s) to Queue__JKI_lib_State_Machine.vi"("State(s) in (\"\")"=w264) -> ("States Out"=w263:string)  [unwired: 14 in]
      }
      frame "Action: Update Channels List" {
        n103 = Unbundle By Name(w270) -> ("Channels ref"=w268:refnum<vi>, "Calibration Data"=w269:T4[])
        n104 = for {
          tunnel: w269 -> [w276] mode=indexing
          tunnel: [w273] -> w267 mode=indexing
          n105 = Unbundle By Name(w276) -> ("Name"=w275:string, "Tag"=w274)
          n106 = Build Array(w275, w274) -> (w273:string[])
        }
        n107 = property class="MCListbox (strict)"(reference=w268, error in=w266, "ItemNames"=w267) -> (error out=w265:errorcluster)  [unwired: 1 out]
        n108 = call <vilib>:"Add State(s) to Queue__JKI_lib_State_Machine.vi"("State(s) in (\"\")"=w272) -> ("States Out"=w271:string)  [unwired: 14 in]
      }
      frame "Action: Update Calibration Tbl" {
        n109 = Unbundle By Name(w285) -> ("Channels config ref"=w284:refnum<vi>, "Calibration Data"=w281:T4[], "Channels"=w280:i32)
        n110 = Index Array(array=w281, index=w280) -> (element=w279:T4)
        n111 = Unbundle By Name(w279) -> ("Calibration"=w278)
        n112 = for {
          tunnel: w278 -> [w293]
          tunnel: [w292] -> w277 mode=indexing
          n113 = Unbundle By Name(w293) -> ("RAW"=w291, "SCL"=w290)
          n114 = Number To Fractional String(number=w291) -> (F-format string=w289:string)  [unwired: 3 in]
          n115 = Number To Fractional String(number=w290) -> (F-format string=w288:string)  [unwired: 3 in]
          n116 = Build Array(w289, w288) -> (w292:string[])
        }
        n117 = property class="MCListbox (strict)"(reference=w284, error in=w283, "ItemNames"=w277) -> (error out=w282:errorcluster)  [unwired: 1 out]
        n118 = call <vilib>:"Add State(s) to Queue__JKI_lib_State_Machine.vi"("State(s) in (\"\")"=w287) -> ("States Out"=w286:string)  [unwired: 14 in]
      }
      frame "Action: Update Calib Graph" {
        n119 = Unbundle By Name(w298) -> ("Calibration Data"=w297:T4[], "Channels"=w296:i32)
        n120 = in-place {
          w303 = T7 0 items=["Least Square", "Least Absolute Residual", "Bisquare"] ("method")
          n121 = in-place-array #7(w297, w296) -> (w309:T4)
          n122 = Unbundle By Name(w309) -> ("Calibration"=w312)
          n123 = for {
            tunnel: w312 -> [w315]
            tunnel: [w314] -> w307 mode=indexing
            tunnel: [w313] -> w310 mode=indexing
            n124 = Unbundle By Name(w315) -> ("RAW"=w314, "SCL"=w313)
          }
          n125 = call <vilib>:"Linear Fit.vi"("Y"=w310, "X"=w307, "method"=w303) -> ("Best Linear Fit"=w306:dbl[], "slope"=w301:dbl, "intercept"=w302:dbl)  [unwired: 8 in, 2 out]
          "Коэфициент усиление" <- w301
          "Offset" <- w302
          n126 = Bundle(w307, w310) -> (w304:cluster{void[], void[]})  [unwired: 1 in]
          n127 = Bundle(cluster=w304, w306) -> (w305:cluster{void[], void[]})  [unwired: 1 in]
          n128 = Build Array(w304, w305) -> (→"XY Graph - Dark":cluster{void[], void[]}[])
          n129 = Bundle By Name(cluster=w309, "k"=w301, "offset"=w302) -> (w308:T4)
          n130 = in-place-array #7(w308) -> (w294:T4[])  [unwired: 1 out]
        }
        n131 = Bundle By Name(cluster=w298, "Calibration Data"=w294) -> (w295:T5)
      }
      frame "Action: 2" {
        # "Your code here.\n(You can make a copy of, or modify, this frame)"
        n132 = call <vilib>:"Add State(s) to Queue__JKI_lib_State_Machine.vi"("State(s) in (\"\")"=w319) -> ("States Out"=w318:string)  [unwired: 14 in]
      }
    }
  }
  "error out" <- w1
